vi "ForceControlIR.vi"() -> ()   [LabVIEW 2015]
uses:
  <vilib>/Platform/TimedLoop/XDataNode/timing_clust.ctl
  <vilib>/Platform/TimedLoop/XDataNode/nitl_modes.ctl
  <vilib>/Platform/TimedLoop/XDataNode/wakeup.ctl
  <vilib>/myRIO/Instrument Drivers/Onboard IO/AI/typedefs/AI Reference.ctl
  <vilib>/myRIO/Common/Instrument Driver Framework/Utilities/typedefs/myRIO Generic Hardware Reference.ctl
  <vilib>/myRIO/Common/Instrument Driver Framework/Utilities/typedefs/Hardware Version Enum.ctl
  <vilib>/myRIO/Common/Instrument Driver Framework/Utilities/typedefs/myRIO v1.0 Reference.ctl
  <vilib>/myRIO/Common/Instrument Driver Framework/Utilities/typedefs/Generic FPGA Reference.ctl
  <vilib>/myRIO/Common/Instrument Driver Framework/myRIO v1.0/AI/typedefs/AI Channels List.ctl
  <vilib>/myRIO/Common/Instrument Driver Framework/myRIO v1.0/AI/typedefs/AI Channels Enum.ctl
  <vilib>/myRIO/Common/Instrument Driver Framework/Utilities/typedefs/Analog Scaling Constants List.ctl
  <vilib>/myRIO/Common/Instrument Driver Framework/Utilities/typedefs/Analog Scaling Constants.ctl
  <vilib>/userdefined/High Color/nirio_resource_hc.ctl
  <vilib>/myRIO/Instrument Drivers/Onboard IO/AO/typedefs/AO Reference.ctl
  <vilib>/myRIO/Common/Instrument Driver Framework/myRIO v1.0/AO/typedefs/AO Channels List.ctl
  <vilib>/myRIO/Common/Instrument Driver Framework/myRIO v1.0/AO/typedefs/AO Channels Enum.ctl
  <vilib>/myRIO/Common/Instrument Driver Framework/Utilities/vis/Is FPGA Ref Available.vi
  <vilib>/myRIO/Common/Instrument Driver Framework/myRIO v1.0/AI/vis/myRIO v1.1 Open AI.vi
  <vilib>/myRIO/Instrument Drivers/Onboard IO/AI/vis/Read.vi
  <vilib>/myRIO/Common/Instrument Driver Framework/myRIO v1.0/AO/vis/myRIO v1.1 Open AO.vi
  <vilib>/myRIO/Instrument Drivers/Onboard IO/AO/vis/Write.vi
  <vilib>/myRIO/Common/Instrument Driver Framework/Utilities/vis/Validate Channels.vi
  <vilib>/myRIO/Common/Instrument Driver Framework/myRIO v1.0/AI/vis/myRIO v1.0 Reserve AI.vi
  <vilib>/myRIO/Common/Instrument Driver Framework/myRIO v1.0/AO/vis/myRIO v1.0 Reserve AO.vi
  <vilib>/myRIO/Common/Instrument Driver Framework/myRIO v1.0/UART/vis/myRIO v1.0 Close UART.vi
  <vilib>/myRIO/Common/Instrument Driver Framework/myRIO v1.0/AI/vis/myRIO v1.0 Build MUX Configuration AI.vi
  <vilib>/myRIO/Common/Instrument Driver Framework/myRIO v1.0/Resource Manager/vis/myRIO v1.0 Reserve Channel List.vi
  <vilib>/myRIO/Common/Instrument Driver Framework/myRIO v1.0/AO/vis/myRIO v1.0 Build MUX Configuration AO.vi
  <vilib>/myRIO/Common/Instrument Driver Framework/myRIO v1.0/Resource Manager/vis/myRIO v1.0 Reserve Channel.vi
  <vilib>/myRIO/Common/Instrument Driver Framework/myRIO v1.0/Resource Manager/vis/myRIO v1.0 Unreserve Channel.vi
  <vilib>/myRIO/Common/Instrument Driver Framework/myRIO v1.0/Resource Manager/vis/myRIO v1.0 Build Mutex Name.vi
  <vilib>/Utility/VariantDataType/GetNumericInfo.vi
  <vilib>/Utility/error.llb/Error Cluster From Error Code.vi
  <vilib>/myRIO/Common/Instrument Driver Framework/myRIO v1.0/myRIO v1.1 Open.vi
  <vilib>/myRIO/Common/Instrument Driver Framework/myRIO v1.0/AI/vis/myRIO v1.0 Get Scaling Constants AI.vi
  <vilib>/myRIO/Common/Instrument Driver Framework/Utilities/vis/IO Manager.vi
  <vilib>/myRIO/Common/Instrument Driver Framework/Utilities/vis/Configuration Manager.vi
  <vilib>/myRIO/Common/Instrument Driver Framework/myRIO v1.0/myRIO v1.0 Close.vi
  <vilib>/myRIO/Common/Instrument Driver Framework/myRIO v1.0/AI/vis/myRIO v1.0 Read AI.vi
  <vilib>/myRIO/Common/Instrument Driver Framework/myRIO v1.0/AO/vis/myRIO v1.0 Get Scaling Constants AO.vi
  <vilib>/myRIO/Common/Instrument Driver Framework/myRIO v1.0/AO/vis/myRIO v1.0 Write AO.vi
  <vilib>/myRIO/Common/Instrument Driver Framework/Utilities/vis/FPGA Ref Manager.vi
  <vilib>/myRIO/Common/Instrument Driver Framework/myRIO v1.0/myRIO v1.0 Reset FPGA.vi
  <vilib>/myRIO/Common/Instrument Driver Framework/myRIO v1.0/IRQ/vis/myRIO v1.0 IRQ Info FGV.vi
  <vilib>/myRIO/Common/Instrument Driver Framework/myRIO v1.0/IRQ/vis/myRIO v1.0 Timer IRQ Info FGV.vi
  <vilib>/myRIO/Common/Instrument Driver Framework/myRIO v1.0/IRQ/vis/myRIO v1.0 ISR Agent.vi
  <vilib>/platform/TimedLoop/XDataNode/XDataNode.xnode
  <vilib>/myRIO/Express VI/Onboard IO/AI/AI Express VI.xnode
  <vilib>/myRIO/Instrument Drivers/Onboard IO/AI/vis/myRIO AI Open.xnode
  <vilib>/myRIO/Express VI/Onboard IO/AO/AO Express VI.xnode
  <vilib>/myRIO/Instrument Drivers/Onboard IO/AO/vis/myRIO AO Open.xnode
  <vilib>/myRIO/Instrument Drivers/Utilities/Utilities.lvlib
  <vilib>/Platform/TimedLoop/XDataNode/XDNodeRunTimeDep.lvlib
  <vilib>/myRIO/Instrument Drivers/Onboard IO/AI/AI.lvlib
  <vilib>/myRIO/Instrument Drivers/Onboard IO/AO/AO.lvlib
panel:
  in  "KiForce":dbl
  in  "Reference Force":dbl
  in  "Ki'":dbl
  in  "Kd'":dbl
  in  "Kp":dbl
  out "Waveform \nChart":dbl(graph)
  in  "stop":bool
  in  "Gripper\nOpening in mm":dbl
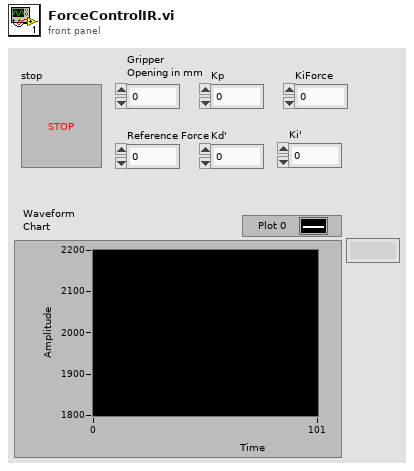
[diagram p1: front panel]
types:
  T1 = typedef "XDNodeRunTimeDep.lvlib/timing_clust.ctl" = cluster{"Expected End [f-1]":u64, "Actual End [f-1]":u64, "Finished Late? [f-1]":bool, "Expected End [i-1]":u64, "Actual End [i-1]":u64, "Finished Late? [i-1]":bool, "Expected Start [i]":u64, "Actual Start [i]":u64, "Expected Start [f]":u64, "Actual Start [f]":u64, "Source Name":string, "Structure Name":string, "Period":i64, "Deadline":i64, "Offset":i64, "Start":i64, "Priority":i32, "Timeout":i32, "Mode":T2, "Wakeup Reason":T3, "Error":errorcluster, "Source Type":string, "Secondary Source Type":string, "Global End Time":u64, "Global Start Time":u64, "Frame Duration":u64, "Iteration Duration":u64, "Assigned CPU":i32, "I/O Scan Engine Mode":u32}
  T2 = typedef "XDNodeRunTimeDep.lvlib/nitl_modes.ctl" = enum32{"No Change", "Process missed periods, maintain original phase", "Discard missed periods, maintain original phase", "Process missed periods, ignore original phase", "Discard missed periods, ignore original phase"}
  T3 = typedef "XDNodeRunTimeDep.lvlib/wakeup.ctl" = enum32{"Normal", "Aborted", "Asynchronous wakeup", "Timing source error", "Timed loop error", "Timeout"}
  T4 = typedef "AI.lvlib/AI Reference.ctl" = cluster{"myRIO Reference":T5, "AI Channels List":T9, "AI Scaling Constants List":T11}
  T5 = typedef "myRIO Generic Hardware Reference.ctl" = cluster{"myRIO Model":T6, "myRIO Hardware Reference":T7}
  T6 = typedef "Hardware Version Enum.ctl" = enum16{"Unknown", "myRIO-1900", "myRIO-1950", "roboRIO"}
  T7 = typedef "myRIO v1.0 Reference.ctl" = cluster{"Generic FPGA Reference":T8, "Allow multiple opens":bool}
  T8 = typedef "Generic FPGA Reference.ctl" = refnum<k20>
  T9 = typedef "AI Channels List.ctl" = T10[]
  T10 = typedef "AI Channels Enum.ctl" = enum16{"Not Connected", "AudioIn/Left", "AudioIn/Right", "C/AI0", "C/AI1", "A/AI0", "A/AI1", "A/AI2", "A/AI3", "B/AI0", "B/AI1", "B/AI2", "B/AI3", "AI/AI0", "AI/AI1", "AI/AI2", "AI/AI3"}
  T11 = typedef "Analog Scaling Constants List.ctl" = T12[]
  T12 = typedef "Analog Scaling Constants.ctl" = cluster{"LSB Weight (Volts)":dbl, "Offset (Volts)":dbl, "Signed?":bool}
  T13 = typedef "nirio_resource_hc.ctl" = tag
  T14 = typedef "AO.lvlib/AO Reference.ctl" = cluster{"myRIO Reference":T5, "AO Channel List":T15, "AO Scaling Constant List":T11}
  T15 = typedef "AO Channels List.ctl" = T16[]
  T16 = typedef "AO Channels Enum.ctl" = enum16{"Not Connected", "AudioOut/Left", "AudioOut/Right", "C/AO0", "C/AO1", "A/AO0", "A/AO1", "B/AO0", "B/AO1"}
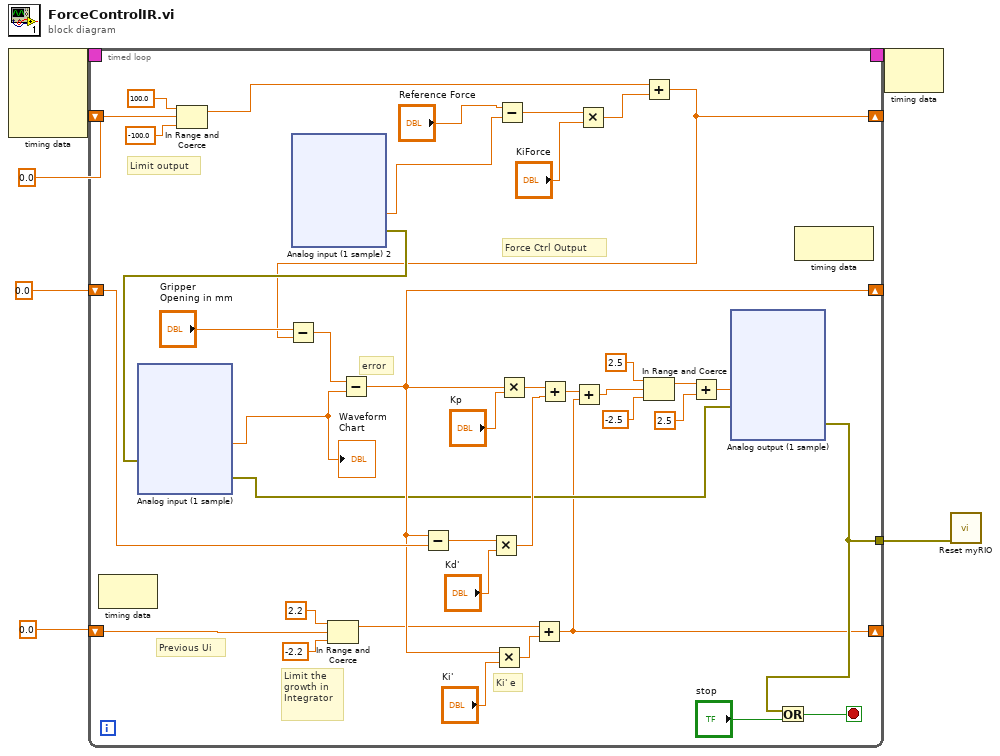
[diagram p0: block diagram]
diagram:
  n1 = node-c288() -> (w5:T1)  [unwired: 4 in]
  n2 = timed-loop {
    tunnel: [w39] -> w6
    timing: w5 -> [_]
    timing-out: [_] -> w4
    shift-right: [w32] -> _
    shift-left: 0.0 -> [w36]
    shift-right: [w11] -> _
    shift-left: 0.0 -> [w26]
    shift-right: [w10] -> _
    shift-left: 0.0 -> [w17]
    stop <- w40 stop-if-true
    # "Limit output"
    # "Force Ctrl Output"
    # "Limit the\ngrowth in\nIntegrator"
    # "Previous Ui"
    # "Ki' e"
    # "error"
    n3 = node-c288() -> ()  [unwired: 1 in, 1 out]
    n4 = In Range and Coerce(upper limit=100.0, x=w17, lower limit=-100.0) -> (coerced(x)=w13:dbl)  [unwired: 1 out]
    n5 = xnode "Analog input (1 sample) 2"() -> ("B/AI1 (Pin 5)"=w8:dbl, "error out"=w20:errorcluster)  [unwired: 1 in]
    n6 = xnode "Analog input (1 sample)"("error in (no error)"=w20) -> ("B/AI0 (Pin 3)"=w9:dbl, "error out"=w23:errorcluster)
    "Waveform \nChart" <- w9
    n7 = In Range and Coerce(upper limit=2.2, x=w26, lower limit=-2.2) -> (coerced(x)=w27:dbl)  [unwired: 1 out]
    n8 = Subtract(x="Reference Force", y=w8) -> (x-y=w19:dbl)
    n9 = Multiply(x=w19, y="KiForce") -> (x*y=w12:dbl)
    n10 = Add(x=w13, y=w12) -> (x+y=w10:dbl)
    n11 = Subtract(x="Gripper\nOpening in mm", y=w10) -> (x-y=w21:dbl)
    n12 = Subtract(x=w21, y=w9) -> (x-y=w32:dbl)
    n13 = Subtract(x=w32, y=w36) -> (x-y=w35:dbl)
    n14 = Multiply(x=w35, y="Kd'") -> (x*y=w33:dbl)
    n15 = Multiply(x=w32, y="Ki'") -> (x*y=w30:dbl)
    n16 = Multiply(x=w32, y="Kp") -> (x*y=w37:dbl)
    n17 = Add(x=w27, y=w30) -> (x+y=w11:dbl)
    n18 = Add(x=w37, y=w33) -> (x+y=w29:dbl)
    n19 = Add(x=w29, y=w11) -> (x+y=w28:dbl)
    n20 = In Range and Coerce(upper limit=2.5, x=w28, lower limit=-2.5) -> (coerced(x)=w43:dbl)  [unwired: 1 out]
    n21 = Add(x=w43, y=2.5) -> (x+y=w7:dbl)
    n22 = xnode "Analog output (1 sample)"("B/AO0 (Pin 2)"=w7, "error in (no error)"=w23) -> ("error out"=w39:errorcluster)
    n23 = Or(x=w39, y="stop") -> (x .or. y?=w40:bool)
    n24 = node-c288() -> ()  [unwired: 1 in, 1 out]
  }
  n25 = node-c288(w4) -> ()  [unwired: 1 out]
  n26 = call <vilib>:"Reset myRIO.vi"("error in (no error)"=w6) -> ()  [unwired: 10 in, 1 out]
